vi "iWorx - Microphone.vi"() -> ()   [LabVIEW 2012]
uses:
  <vilib>/DAQmx/read.llb/DAQmx Read (Analog 1D Wfm NChan NSamp).vi
  <vilib>/DAQmx/create/channels.llb/DAQmx Create Channel (AI-Voltage-Basic).vi
  <vilib>/DAQmx/configure/timing.llb/DAQmx Timing (Sample Clock).vi
  <vilib>/DAQmx/miscellaneous.llb/DAQmx Fill In Error Info.vi
panel:
  in  "Set Up":bool
  in  "Channel":enum16{"Right", "Left", "Both"}(ring)
  in  "Pause Button":bool
  in  "Snapshot":bool
  in  "stop":bool
  out "Waveform Chart":waveform(dbl)[](graph)
  in  "Clear Chart":bool
  in  "Open Log":bool
  in  "Autoscale Y":bool
  # "iWorx - Microphone - Data Logger"
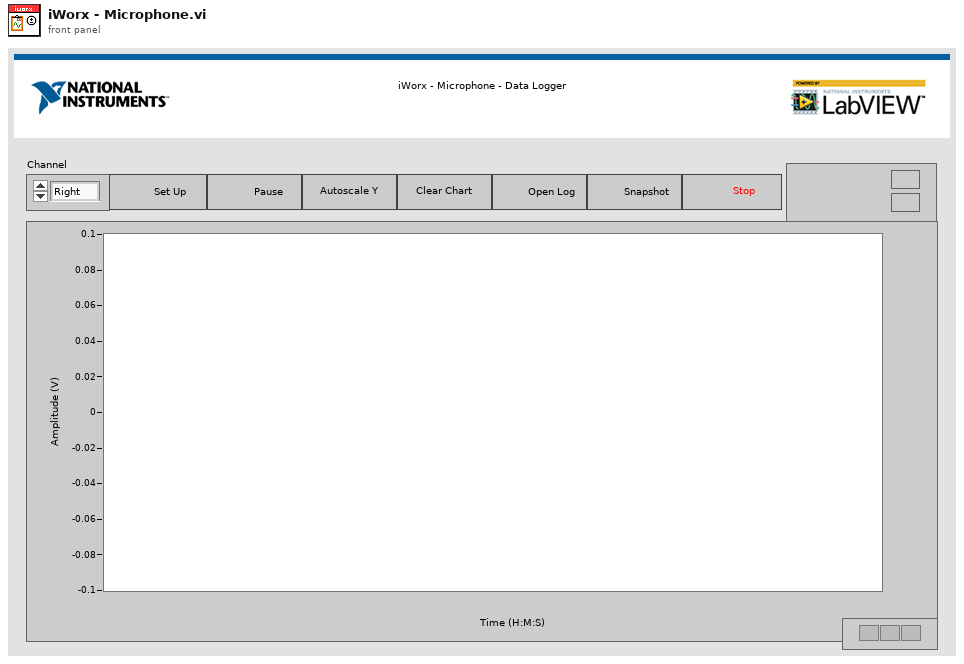
[diagram p1: front panel]
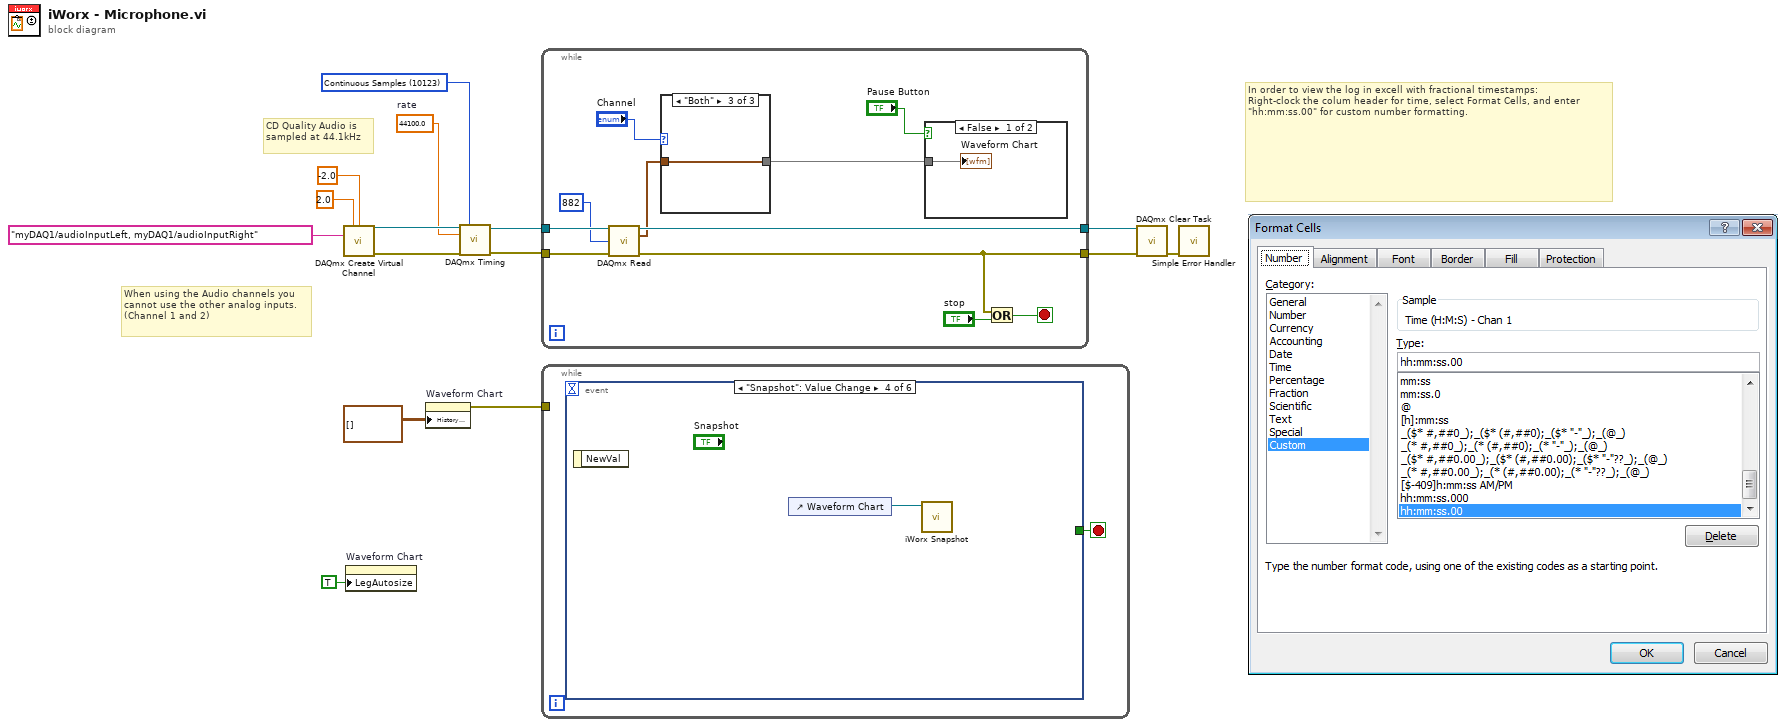
[diagram p0: block diagram]
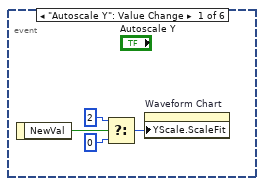
[diagram p2: hidden frame]
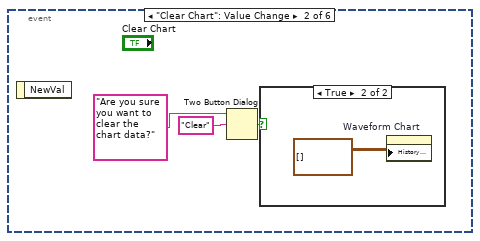
[diagram p3: hidden frame]
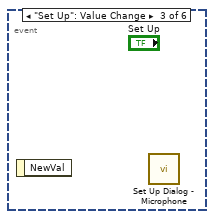
[diagram p5: hidden frame]
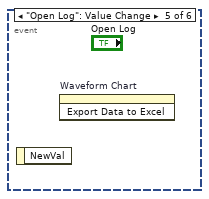
[diagram p6: hidden frame]
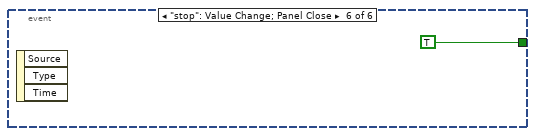
[diagram p7: hidden frame]
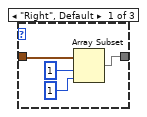
[diagram p8: hidden frame]
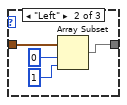
[diagram p9: hidden frame]
diagram:
  w5 = 44100.0  # rate
  w6 = 10123 items=["Finite Samples"=10178, "Continuous Samples"=10123, "Hardware Timed Single Point"=12522] ("sample mode")
  # "When using the Audio channels you cannot use the other analog inputs. (Channel 1 and 2)"
  # "CD Quality Audio is sampled at 44.1kHz"
  # "In order to view the log in excell with fractional timestamps: \nRight-clock the colum header for time, select Format Cells, and enter \"hh:mm:ss.00\" for custom number formatting."
  n1 = call-poly <vilib>:"DAQmx Create Virtual Channel.vi"("maximum value"=2.0, "minimum value"=-2.0, "physical channels"=tag "myDAQ1/audioInputLeft, myDAQ1/audioInputRight") -> ("task out"=w10:refnum<k21>, "error out"=w9:errorcluster)  [unwired: 11 in]
  n2 = property on="Waveform Chart" class="WFChart (strict)"("LegAutosize"=TRUE ("Legend:Autosize")) -> ()  [unwired: 2 in, 2 out]
  n3 = property on="Waveform Chart" class="WFChart (strict)"("History Data"=waveform(dbl)[][] []) -> (error out=w12:errorcluster)  [unwired: 2 in, 1 out]
  n4 = call-poly <vilib>:"DAQmx Timing.vi"("task/channels in"=w10, "sample mode"=w6, "rate"=w5, "error in"=w9) -> ("task out"=w7:refnum<k21>, "error out"=w8:errorcluster)  [unwired: 10 in]
  n5 = while {
    tunnel: w7 -> [w25]
    tunnel: [w24] -> w15
    tunnel: w8 -> [w23]
    tunnel: [w21] -> w14
    stop <- w22 stop-if-true
    n6 = call-poly <vilib>:"DAQmx Read.vi"("task/channels in"=w25, "number of samples per channel"=882 ("samples per channel"), "error in"=w23) -> ("task out"=w24:refnum<k21>, "data"=w18:waveform(dbl)[], "error out"=w21:errorcluster)  [unwired: 10 in]
    n7 = case shown="\"Both\"" "Channel" {
      tunnel: w18 -> [w28 w34 w35]
      tunnel: [w27 w33 w35] -> w16
      frame "Right", Default {
        n8 = Array Subset(array=w28, index=1, length=1) -> (w27:waveform(dbl)[])
      }
      frame "Left" {
        n9 = Array Subset(array=w34, index=0, length=1) -> (w33:waveform(dbl)[])
      }
      frame "Both" {
      }
    }
    n10 = case shown="False" "Pause Button" {
      tunnel: w16 -> [w36 _]
      frame False {
        "Waveform Chart" <- w36
      }
      frame True {
      }
    }
    n11 = Or(x=w21, y="stop") -> (x .or. y?=w22:bool)
  }
  n12 = while {
    tunnel: w12 -> [_]
    stop <- w37 stop-if-true
    n13 = event shown="[3] \"Snapshot\": Value Change" {
      selector: _ -> [_ _ _ _ _ _]
      dyn-events: _ -> [_ _ _ _ _ _]
      timeout: _ -> [_ _ _ _ _ _]
      tunnel: [_ _ _ _ _ TRUE] -> w37
      event "Autoscale Y": Value Change {
        n14 = event-data() -> ("NewVal"=w39:bool)  [unwired: 1 in]
        n15 = Select(t=u8 2 ("Y Scale.Scale Fit"), s=w39, f=u8 0 ("Y Scale.Scale Fit")) -> (s? t:f=w38:u8)
        n16 = property on="Waveform Chart" class="WFChart (strict)"("YScale.ScaleFit"=w38) -> ()  [unwired: 2 in, 2 out]
      }
      event "Clear Chart": Value Change {
        n17 = event-data() -> ()  [unwired: 1 in, 1 out]
        n18 = Two Button Dialog(message="Are you sure you want to clear the chart data?", 2:"Clear" ("T button name (\"OK\")")) -> (T button?=w43:bool)  [unwired: 1 in]
        n19 = case shown="True" w43 {
          frame False {
          }
          frame True {
            n20 = property on="Waveform Chart" class="WFChart (strict)"("History Data"=waveform(dbl)[][] []) -> ()  [unwired: 2 in, 2 out]
          }
        }
      }
      event "Set Up": Value Change {
        n21 = event-data() -> ()  [unwired: 1 in, 1 out]
        n22 = call "Set Up Dialog - Microphone.vi"() -> ()  [unwired: 12 in]
      }
      event "Snapshot": Value Change {
        n23 = event-data() -> ()  [unwired: 1 in, 1 out]
        n24 = control-ref of="Waveform Chart"() -> (w46:refnum<vi>)
        n25 = call "iWorx Snapshot.vi"("WaveformChart in"=w46) -> ()  [unwired: 10 in, 1 out]
      }
      event "Open Log": Value Change {
        n26 = event-data() -> ()  [unwired: 1 in, 1 out]
        n27 = invoke on="Waveform Chart" class="WFChart (strict)" method="Export Data to Excel"() -> ()  [unwired: 3 in, 3 out]
      }
      event "stop": Value Change; Panel Close {
        n28 = event-data() -> ()  [unwired: 1 in, 3 out]
      }
    }
  }
  n29 = call <vilib>:"DAQmx Clear Task.vi"("task in"=w15, "error in"=w14) -> ("error out"=w11:errorcluster)  [unwired: 13 in]
  n30 = call <vilib>:"Simple Error Handler.vi"("error in (no error)"=w11) -> ()  [unwired: 4 in, 5 out]
